vi "Writer.vi"   [LabVIEW 2020, in "Global_logger.lvlib"]
uses:
  Global_logger.lvlib
  <vilib>/Utility/error.llb/DialogType.ctl
  Logger Output.ctl
  Levels.ctl
  Level Meaning.ctl
  Sorting.ctl
  Logger Type.ctl
  Log Fields.ctl
types:
  T1 = typedef "Global_logger.lvlib/Logger Output.ctl" = cluster{"Level":T2, "Level Meaning":T3, "Sorting":T4, "Type":T5, "Filetype":string, "Filename":string, "Root path":path, "Max filesize (bytes)":i32, "Max age (days)":i32, "Ctl Refnum":refnum<vi>, "String Ctl Delimiter":string, "Format":T6[], "Timestamp format":string}
  T2 = typedef "Global_logger.lvlib/Levels.ctl" = enum16{"ALL", "TRACE", "DEBUG", "INFO", "WARN", "ERROR", "FATAL", "OFF"}
  T3 = typedef "Global_logger.lvlib/Level Meaning.ctl" = enum16{"Standard", "Positive", "Exact"}
  T4 = typedef "Global_logger.lvlib/Sorting.ctl" = enum16{"Add to Bottom", "Add to Top"}
  T5 = typedef "Global_logger.lvlib/Logger Type.ctl" = enum16{"FILE", "UI"}
  T6 = typedef "Global_logger.lvlib/Log Fields.ctl" = enum16{"Timestamp", "Level", "Message", "Source VI", "Source App", "Logger Name"}
  T7 = typedef "DialogType.ctl" = u16
  T8 = typedef "Global_logger.lvlib/Event.ctl" = cluster{"Logger Name":string, "Time Stamp":timestamp, "Level":T2, "Source VI":string, "Message":string, "Source App":string}
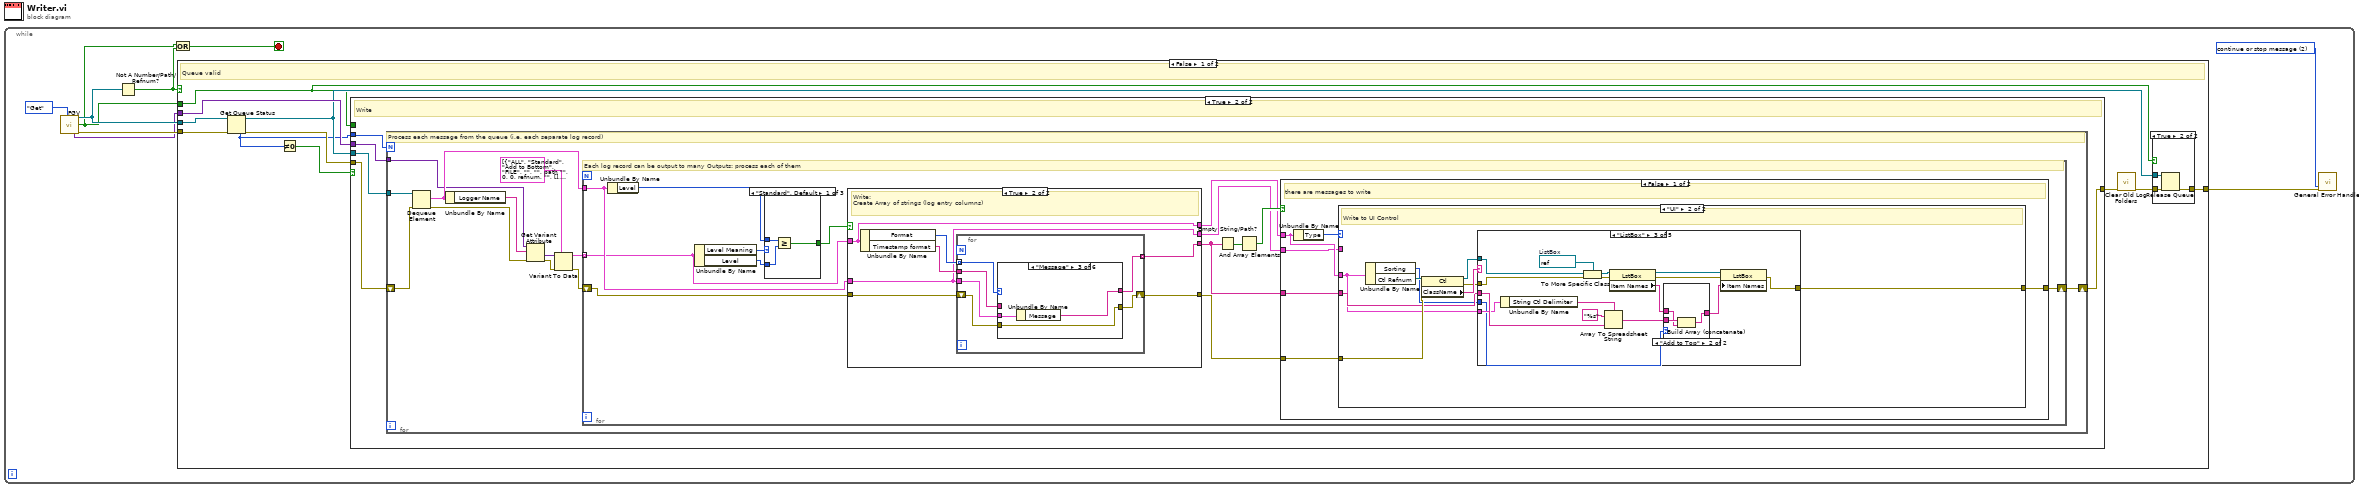
[diagram p0: block diagram]
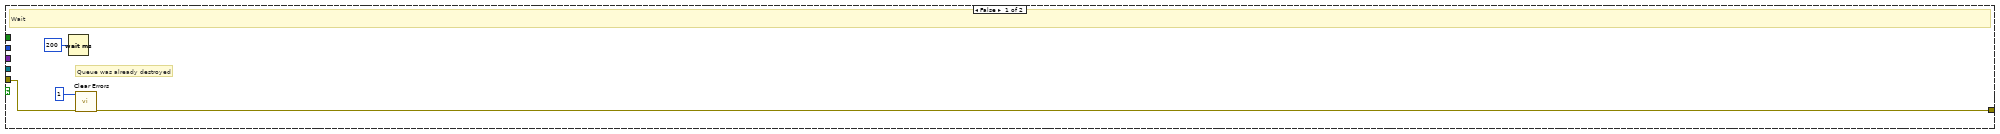
[diagram p3: hidden frame]
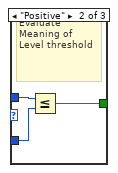
[diagram p4: hidden frame]
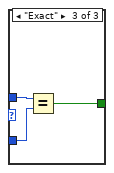
[diagram p5: hidden frame]
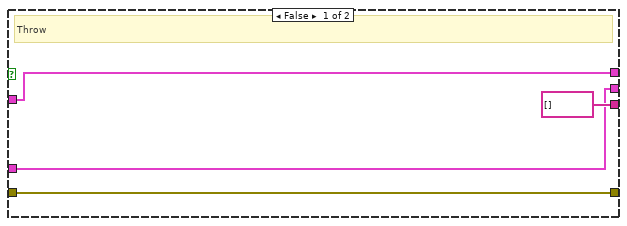
[diagram p6: hidden frame]
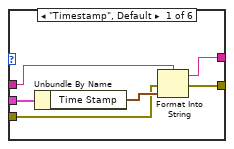
[diagram p7: hidden frame]
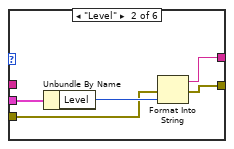
[diagram p8: hidden frame]
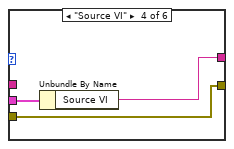
[diagram p9: hidden frame]
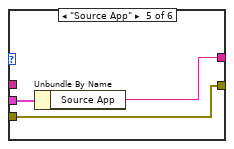
[diagram p10: hidden frame]
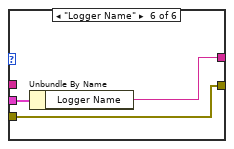
[diagram p11: hidden frame]
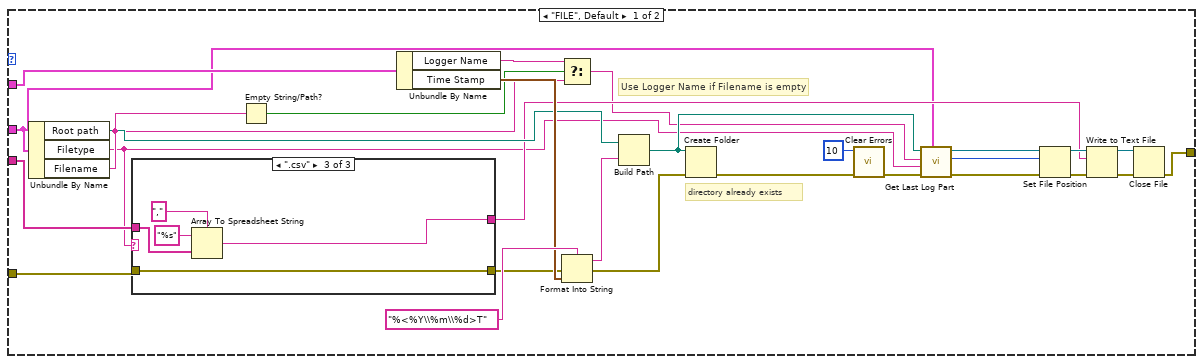
[diagram p12: hidden frame]
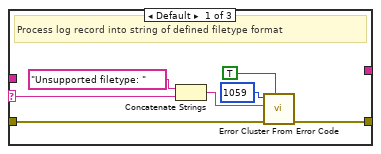
[diagram p13: hidden frame]
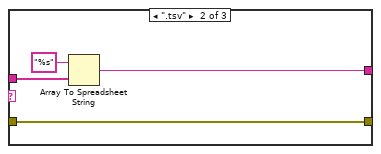
[diagram p14: hidden frame]
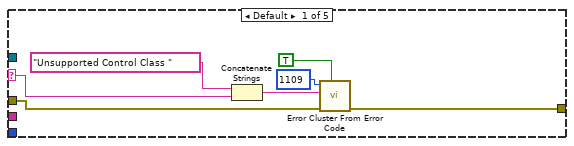
[diagram p15: hidden frame]
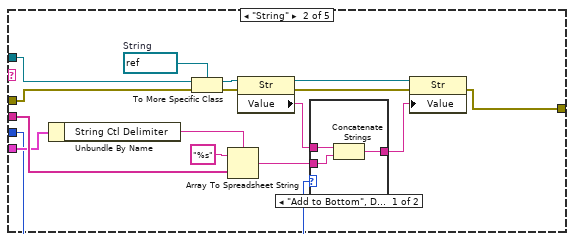
[diagram p16: hidden frame]
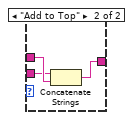
[diagram p17: hidden frame]
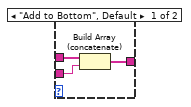
[diagram p18: hidden frame]
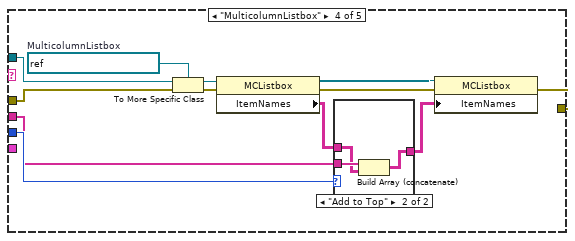
[diagram p19: hidden frame]
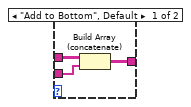
[diagram p20: hidden frame]
diagram:
  n1 = while {
    stop <- w4 stop-if-true
    w5 = T7 2 items=["no dialog", "OK message", "continue or stop message", "OK message + warnings", "continue/stop + warnings"] ("type of dialog (OK msg:1)")
    n2 = call "FGV.vi"("Action"=enum16{"Get", "Set"}."Get") -> ("queue out"=w6:refnum<queue>, "Destroy Logger out"=w2:bool, "All Named Loggers"=w1:variant, "error out"=w8:errorcluster)  [unwired: 9 in, 2 out]
    n3 = Not A Number/Path/Refnum?(number/path/refnum=w6) -> (NaN/Path/Refnum?=w3:bool)
    n4 = Or(x=w2, y=w3) -> (x .or. y?=w4:bool)
    n5 = case shown="False" w3 {
      tunnel: w8 -> [w10 _]
      tunnel: w1 -> [w19 _]
      tunnel: [w18 _] -> w7
      tunnel: w2 -> [w11 _]
      tunnel: w6 -> [w12 _]
      frame False {
        # "Queue valid"
        n6 = Get Queue Status(queue=w12, error in (no error)=w10) -> (queue out=w17:refnum<queue>, error out=w20:errorcluster, # elements in queue=w14:i32)  [unwired: 1 in, 5 out]
        n7 = Not Equal To 0?(x=w14) -> (x != 0?=w13:bool)
        n8 = case shown="True" w13 {
          tunnel: w17 -> [_ w33]
          tunnel: w20 -> [w28 w32]
          tunnel: w19 -> [_ w29]
          tunnel: [w27 w31] -> w16
          tunnel: w11 -> [_ _]
          tunnel: w14 -> [_ w30]
          frame False {
            # "Queue was already destroyed"
            # "Wait"
            n9 = Wait (ms)(milliseconds to wait=u32 200) -> ()  [unwired: 1 out]
            n10 = call <vilib>:"Clear Errors.vi"("error in (no error)"=w28, "specific error code to clear (0: all)"=1) -> ("error out"=w27:errorcluster)  [unwired: 4 in, 1 out]
          }
          frame True {
            # "Write"
            n11 = for {
              N: w30 -> [_]
              tunnel: w33 -> [w45]
              shift-right: [w43] -> w31
              shift-left: w32 -> [w44]
              tunnel: w29 -> [w34]
              # "Process each message from the queue (i.e. each separate log record)"
              n12 = Dequeue Element(queue=w45, error in (no error)=w44) -> (element=w36:T8, error out=w42:errorcluster)  [unwired: 1 in, 2 out]
              n13 = Unbundle By Name(w36) -> ("Logger Name"=w35:string)
              n14 = Get Variant Attribute(Variant=w34, name=w35, error in=w42) -> (value=w39:variant, error out=w41:errorcluster)  [unwired: 1 in, 2 out]
              n15 = Variant To Data(error in=w41, type=T1[] [{"Level"=enum."ALL", "Level Meaning"=enum."Standard", "Sorting"=enum."Add to Bottom", "Type"=enum."FILE", "Filetype"="", "Filename"="", "Root path"=path "", "Max filesize (bytes)"=0, "Max age (days)"=0, "Ctl Refnum"=refnum, "String Ctl Delimiter"="", "Format"=[], "Timestamp format"=""}], Variant=w39) -> (data=w37:T1[], error out=w40:errorcluster)
              n16 = for {
                shift-right: [w58] -> w43
                shift-left: w40 -> [w54]
                tunnel: w37 -> [w49] mode=indexing
                tunnel: w36 -> [w51]
                # "Each log record can be output to many Outputs: process each of them"
                n17 = Unbundle By Name(w51) -> ("Level"=w50:T2)
                n18 = Unbundle By Name(w49) -> ("Level Meaning"=w53:T3, "Level"=w52:T2)
                n19 = case shown="\"Standard\", Default" w53 {
                  tunnel: [w62 w63 w66] -> w56
                  tunnel: w50 -> [w61 w65 w68]
                  tunnel: w52 -> [w60 w64 w67]
                  frame "Standard", Default {
                    n20 = Greater Or Equal?(x=w61, y=w60) -> (x >= y?=w62:bool)
                  }
                  frame "Positive" {
                    # "Evaluate Meaning of Level threshold"
                    n21 = Less Or Equal?(x=w65, y=w64) -> (x <= y?=w63:bool)
                  }
                  frame "Exact" {
                    n22 = Equal?(x=w68, y=w67) -> (x = y?=w66:bool)
                  }
                }
                n23 = case shown="True" w56 {
                  tunnel: [string[] [] w75] -> w55
                  tunnel: w54 -> [w72 w78]
                  tunnel: [w72 w76] -> w59
                  tunnel: w51 -> [w69 w73]
                  tunnel: w49 -> [w70 w74]
                  tunnel: [w70 w74] -> w47
                  tunnel: [w69 w73] -> w46
                  frame False {
                    # "Throw"
                  }
                  frame True {
                    # "Write: \nCreate Array of strings (log entry columns)"
                    n24 = Unbundle By Name(w74) -> ("Format"=w79:T6[], "Timestamp format"=w77:string)
                    n25 = for {
                      tunnel: w79 -> [w85] mode=indexing
                      tunnel: w73 -> [w84]
                      tunnel: w77 -> [w81]
                      shift-right: [w82] -> w76
                      shift-left: w78 -> [w83]
                      tunnel: [w80] -> w75 mode=indexing
                      n26 = case shown="\"Message\"" w85 {
                        tunnel: w84 -> [w91 w96 w99 w102 w105 w108]
                        tunnel: w83 -> [w89 w94 w97 w100 w103 w106]
                        tunnel: [w88 w93 w97 w100 w103 w106] -> w82
                        tunnel: [w86 w92 w98 w101 w104 w107] -> w80
                        tunnel: w81 -> [w87 _ _ _ _ _]
                        frame "Timestamp", Default {
                          n27 = Unbundle By Name(w91) -> ("Time Stamp"=w90:timestamp)
                          n28 = Format Into String(format string=w87, error in=w89, w90) -> (resulting string=w86:string, error out=w88:errorcluster)  [unwired: 1 in]
                        }
                        frame "Level" {
                          n29 = Unbundle By Name(w96) -> ("Level"=w95:T2)
                          n30 = Format Into String(error in=w94, w95) -> (resulting string=w92:string, error out=w93:errorcluster)  [unwired: 2 in]
                        }
                        frame "Message" {
                          n31 = Unbundle By Name(w99) -> ("Message"=w98:string)
                        }
                        frame "Source VI" {
                          n32 = Unbundle By Name(w102) -> ("Source VI"=w101:string)
                        }
                        frame "Source App" {
                          n33 = Unbundle By Name(w105) -> ("Source App"=w104:string)
                        }
                        frame "Logger Name" {
                          n34 = Unbundle By Name(w108) -> ("Logger Name"=w107:string)
                        }
                      }
                    }
                  }
                }
                n35 = Empty String/Path?(string/path=w55) -> (empty?=w57:bool[])
                n36 = And Array Elements(Boolean array=w57) -> (logical AND=w48:bool)
                n37 = case shown="False" w48 {
                  tunnel: w59 -> [w114 w255]
                  tunnel: [w113 w255] -> w58
                  tunnel: w55 -> [w112 _]
                  tunnel: w47 -> [w110 _]
                  tunnel: w46 -> [w109 _]
                  frame False {
                    # "there are messages to write"
                    n38 = Unbundle By Name(w110) -> ("Type"=w111:T5)
                    n39 = case shown="\"UI\"" w111 {
                      tunnel: w114 -> [w125 w166]
                      tunnel: [w134 w159] -> w113
                      tunnel: w112 -> [w127 w162]
                      tunnel: w110 -> [w118 w161]
                      tunnel: w109 -> [w132 _]
                      frame "FILE", Default {
                        # "Use Logger Name if Filename is empty"
                        # "directory already exists"
                        n40 = Unbundle By Name(w118) -> ("Root path"=w130:path, "Filetype"=w119:string, "Filename"=w122:string)
                        n41 = case shown="\".csv\"" w119 {
                          selector: w119 -> [w145 _ _]
                          tunnel: w127 -> [_ w153 w158]
                          tunnel: [_ w152 w157] -> w128
                          tunnel: [w144 w151 w155] -> w126
                          tunnel: w125 -> [w143 w151 w155]
                          frame Default {
                            # "Process log record into string of defined filetype format"
                            n42 = Concatenate Strings("Unsupported filetype: " ("error message (\"\")"), w145) -> (w146:string)
                            n43 = call <vilib>:"Error Cluster From Error Code.vi"("show call chain? (False)"=TRUE, "error in (no error)"=w143, "error message (\"\")"=w146, "error code (0)"=1059) -> ("error out"=w144:errorcluster)  [unwired: 5 in]
                          }
                          frame ".tsv" {
                            n44 = Array To Spreadsheet String(array=w153, 3:"%s" ("format string")) -> (spreadsheet string=w152:string)  [unwired: 1 in]
                          }
                          frame ".csv" {
                            n45 = Array To Spreadsheet String(delimiter (Tab)=",", array=w158, 3:"%s" ("format string")) -> (spreadsheet string=w157:string)
                          }
                        }
                        n46 = Empty String/Path?(string/path=w122) -> (empty?=w124:bool)
                        n47 = Unbundle By Name(w132) -> ("Logger Name"=w123:string, "Time Stamp"=w131:timestamp)
                        n48 = Select(t=w123, s=w124, f=w122) -> (s? t:f=w120:string)
                        n49 = Format Into String(format string="%<%Y\\%m\\%d>T", error in=w126, w131) -> (resulting string=w141:string, error out=w140:errorcluster)  [unwired: 1 in]
                        n50 = Build Path(base path=w130, name or relative path=w141) -> (appended path=w129:path)
                        n51 = Create Folder(path (use dialog)=w129, error in=w140) -> (error out=w139:errorcluster)  [unwired: 1 in, 2 out]
                        n52 = call <vilib>:"Clear Errors.vi"("error in (no error)"=w139, "specific error code to clear (0: all)"=10) -> ("error out"=w121:errorcluster)  [unwired: 4 in, 1 out]
                        n53 = call "Get Last Log Part.vi"("Logger Output"=w118, "error in (no error)"=w121, "Filetype"=w119, "Filename"=w120, "Root path in"=w129) -> ("error out"=w116:errorcluster, "File write position"=w117:i64, "File to Write in ref"=w115:refnum<file>)  [unwired: 4 in]
                        n54 = Set File Position(offset (in bytes) (0)=w117, refnum=w115, error in=w116) -> (refnum out=w137:refnum<file>, error out=w136:errorcluster)  [unwired: 1 out]
                        n55 = Write to Text File(file (use dialog)=w137, text=w128, error in=w136) -> (refnum out=w138:refnum<file>, error out=w135:errorcluster)  [unwired: 2 out]
                        n56 = Close File(refnum=w138, error in=w135) -> (error out=w134:errorcluster)  [unwired: 1 out]
                      }
                      frame "UI" {
                        # "Write to UI Control"
                        n57 = Unbundle By Name(w161) -> ("Sorting"=w160:T4, "Ctl Refnum"=w167:refnum<vi>)
                        n58 = property class="Ctl"(reference=w167, error in=w166) -> (reference out=w164:refnum<vi>, error out=w163:errorcluster, "ClassName"=w165:string)
                        n59 = case shown="\"ListBox\"" w165 {
                          selector: w165 -> [w171 _ _ _ _]
                          tunnel: w164 -> [_ w190 w212 w230 w248]
                          tunnel: w163 -> [w169 w189 w211 w229 w247]
                          tunnel: w162 -> [_ w185 w208 w219 w237]
                          tunnel: w161 -> [_ w184 w207 _ _]
                          tunnel: w160 -> [_ w177 w201 w222 w240]
                          tunnel: [w168 w176 w198 w220 w238] -> w159
                          frame Default {
                            n60 = Concatenate Strings("Unsupported Control Class " ("error message (\"\")"), w171) -> (w170:string)
                            n61 = call <vilib>:"Error Cluster From Error Code.vi"("show call chain? (False)"=TRUE, "error in (no error)"=w169, "error message (\"\")"=w170, "error code (0)"=1109) -> ("error out"=w168:errorcluster)  [unwired: 5 in]
                          }
                          frame "String" {
                            w188 = refnum<vi> refnum  # String
                            n62 = Unbundle By Name(w184) -> ("String Ctl Delimiter"=w183:string)
                            n63 = To More Specific Class(target class=w188, reference=w190, error in=w189) -> (specific class reference=w187:refnum<vi>, error out=w186:errorcluster)
                            n64 = Array To Spreadsheet String(delimiter (Tab)=w183, array=w185, 3:"%s" ("format string")) -> (spreadsheet string=w179:string)
                            n65 = property class="Str"(reference=w187, error in=w186) -> (reference out=w182:refnum<vi>, error out=w181:errorcluster, "Value"=w180:string)
                            n66 = case shown="\"Add to Bottom\", Default" w177 {
                              tunnel: w180 -> [w193 w196]
                              tunnel: w179 -> [w192 w195]
                              tunnel: [w191 w194] -> w178
                              frame "Add to Bottom", Default {
                                n67 = Concatenate Strings(w193, w192) -> (w191:string)
                              }
                              frame "Add to Top" {
                                n68 = Concatenate Strings(w195, w196) -> (w194:string)
                              }
                            }
                            n69 = property class="Str"(reference=w182, error in=w181, "Value"=w178) -> (error out=w176:errorcluster)  [unwired: 1 out]
                          }
                          frame "ListBox" {
                            w210 = refnum<vi> refnum  # ListBox
                            n70 = Unbundle By Name(w207) -> ("String Ctl Delimiter"=w206:string)
                            n71 = To More Specific Class(target class=w210, reference=w212, error in=w211) -> (specific class reference=w204:refnum<vi>, error out=w209:errorcluster)
                            n72 = Array To Spreadsheet String(delimiter (Tab)=w206, array=w208, 3:"%s" ("format string")) -> (spreadsheet string=w200:string)
                            n73 = property class="LstBox"(reference=w204, error in=w209) -> (reference out=w203:refnum<vi>, error out=w205:errorcluster, "Item Names"=w199:string[])
                            n74 = case shown="\"Add to Top\"" w201 {
                              tunnel: [w213 w216] -> w202
                              tunnel: w200 -> [w214 w218]
                              tunnel: w199 -> [w215 w217]
                              frame "Add to Bottom", Default {
                                n75 = Build Array (concatenate)(w215, w214) -> (w213:string[])
                              }
                              frame "Add to Top" {
                                n76 = Build Array (concatenate)(w218, w217) -> (w216:string[])
                              }
                            }
                            n77 = property class="LstBox"(reference=w203, error in=w205, "Item Names"=w202) -> (error out=w198:errorcluster)  [unwired: 1 out]
                          }
                          frame "MulticolumnListbox" {
                            w228 = refnum<vi> refnum  # MulticolumnListbox
                            n78 = To More Specific Class(target class=w228, reference=w230, error in=w229) -> (specific class reference=w225:refnum<vi>, error out=w227:errorcluster)
                            n79 = property class="MCListbox"(reference=w225, error in=w227) -> (reference out=w224:refnum<vi>, error out=w226:errorcluster, "ItemNames"=w221:string[][])
                            n80 = case shown="\"Add to Top\"" w222 {
                              tunnel: [w231 w234] -> w223
                              tunnel: w219 -> [w232 w236]
                              tunnel: w221 -> [w233 w235]
                              frame "Add to Bottom", Default {
                                n81 = Build Array (concatenate)(w233, w232) -> (w231:string[][])
                              }
                              frame "Add to Top" {
                                n82 = Build Array (concatenate)(w236, w235) -> (w234:string[][])
                              }
                            }
                            n83 = property class="MCListbox"(reference=w224, error in=w226, "ItemNames"=w223) -> (error out=w220:errorcluster)  [unwired: 1 out]
                          }
                          frame "Table" {
                            w246 = refnum<vi> refnum  # Table
                            n84 = To More Specific Class(target class=w246, reference=w248, error in=w247) -> (specific class reference=w243:refnum<vi>, error out=w245:errorcluster)
                            n85 = property class="Tbl"(reference=w243, error in=w245) -> (reference out=w242:refnum<vi>, error out=w244:errorcluster, "Value"=w239:string[][])
                            n86 = case shown="\"Add to Top\"" w240 {
                              tunnel: [w249 w252] -> w241
                              tunnel: w237 -> [w250 w254]
                              tunnel: w239 -> [w251 w253]
                              frame "Add to Bottom", Default {
                                n87 = Build Array (concatenate)(w251, w250) -> (w249:string[][])
                              }
                              frame "Add to Top" {
                                n88 = Build Array (concatenate)(w254, w253) -> (w252:string[][])
                              }
                            }
                            n89 = property class="Tbl"(reference=w242, error in=w244, "Value"=w241) -> (error out=w238:errorcluster)  [unwired: 1 out]
                          }
                        }
                      }
                    }
                  }
                  frame True {
                    # "no write after all - all messages filtered out"
                  }
                }
              }
            }
          }
        }
        n90 = call "Clear Old Log Folders.vi"("error in (no error)"=w16) -> ("error out"=w15:errorcluster)  [unwired: 10 in]
        n91 = case shown="True" w11 {
          tunnel: [w21 w24] -> w18
          tunnel: w17 -> [_ w23]
          tunnel: w15 -> [w21 w22]
          frame False {
          }
          frame True {
            n92 = Release Queue(queue=w23, error in (no error)=w22) -> (error out=w24:errorcluster)  [unwired: 1 in, 2 out]
          }
        }
      }
      frame True {
        # "Queue invalid"
      }
    }
    n93 = call <vilib>:"General Error Handler.vi"("type of dialog (OK msg:1)"=w5, "error in (no error)"=w7) -> ()  [unwired: 9 in, 5 out]
  }
